vi "전체 Test.vi"() -> ()   [LabVIEW 2020]
uses:
  <vilib>/userDefined/High Color/IMAQdx.ctl
  <vilib>/Utility/miscctls.llb/LVPointTypeDef.ctl
  <vilib>/DAQmx/read.llb/DAQmx Read (Analog 1D Wfm NChan NSamp).vi
  <vilib>/Analysis/baseanly.llb/Mean (DBL).vi
  <vilib>/DAQmx/create/channels.llb/DAQmx Create Channel (AI-Voltage-Basic).vi
  <vilib>/DAQmx/configure/timing.llb/DAQmx Timing (Sample Clock).vi
  <vilib>/DAQmx/miscellaneous.llb/DAQmx Fill In Error Info.vi
  <vilib>/Analysis/NI_AALBase.lvlib
  <vilib>/vision/driver/NI_Vision_Acquisition_Software.lvlib
  <vilib>/Utility/file.llb/Write Delimited Spreadsheet (DBL).vi
panel:
  out "거리":waveform(dbl)(graph)
  out "기울기":waveform(dbl)[](graph)
  out "가속도":waveform(dbl)(graph)
  out "Image":T1(plugin-control)
  in  "data out":string
  out "CNN Result":string[](array[string])
  in  "CNN Data Save Path":path
  out "Capture Image":T1(plugin-control) caption="Captuer Image"
  out "Softmax Result":string
  in  "Softmax Data Save Path":path
  in  "정지":bool
  in  "측정 시작":bool
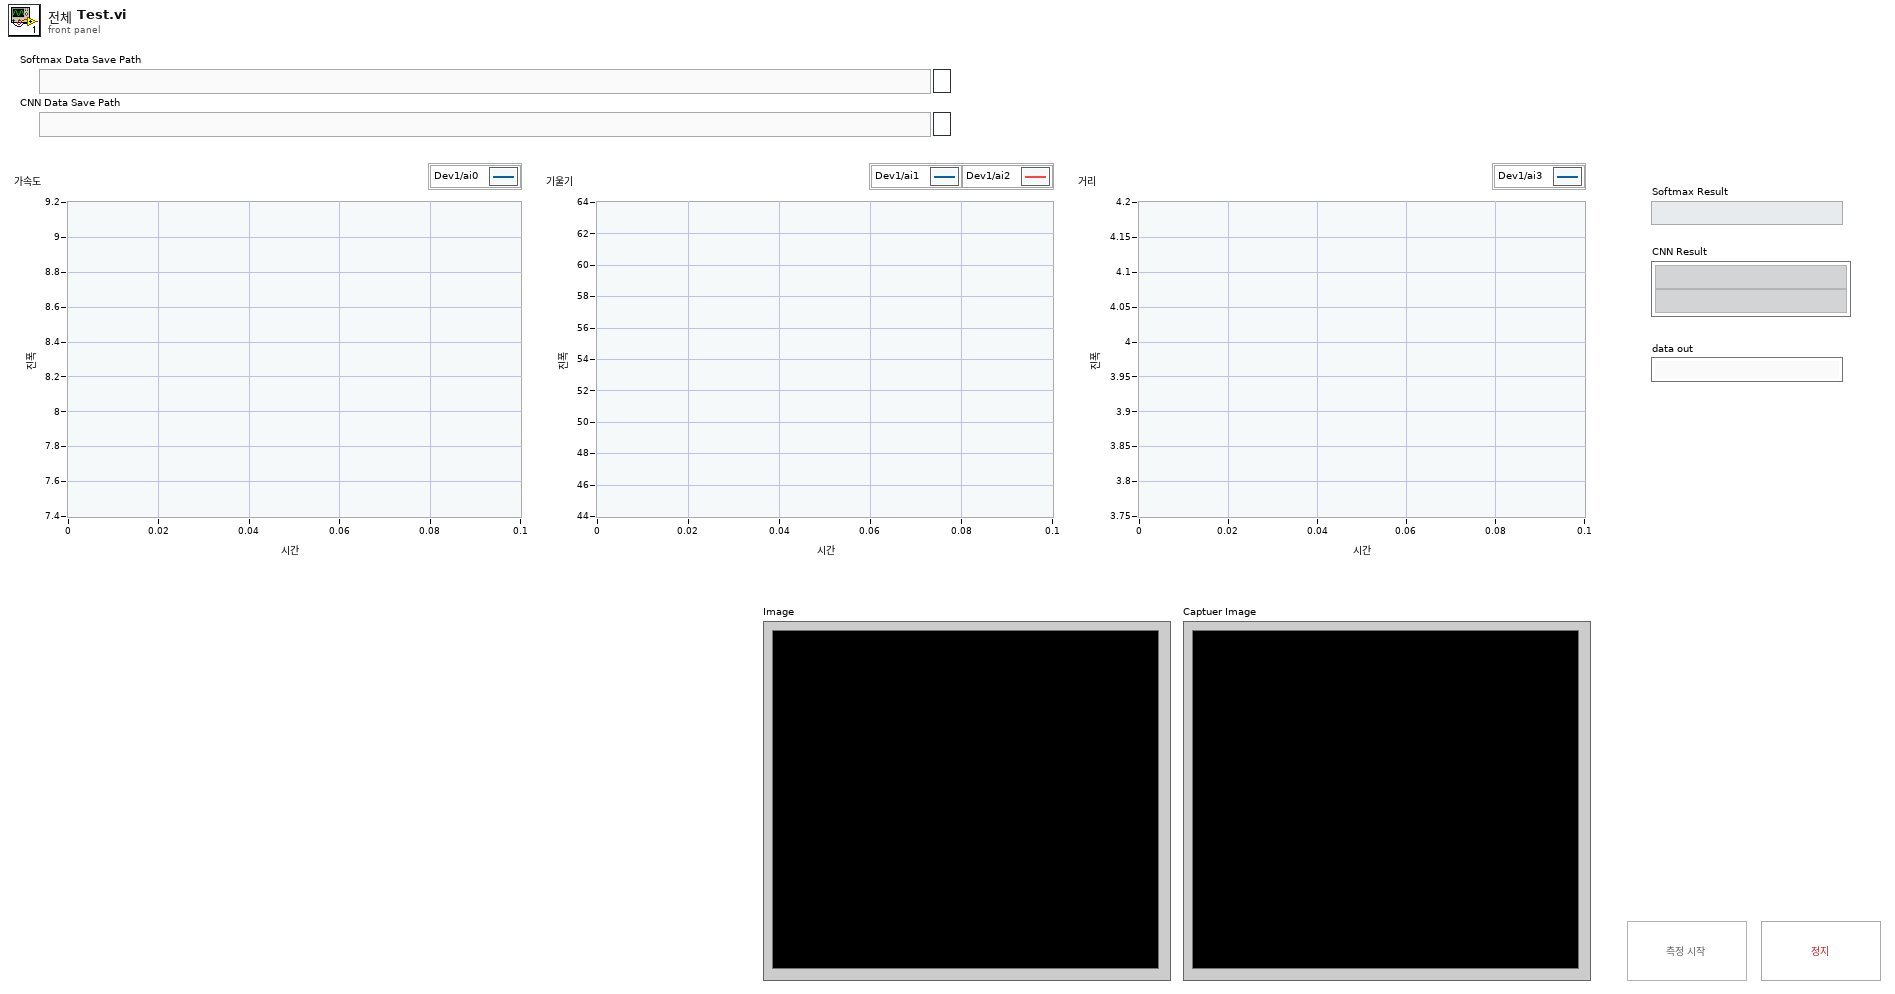
[diagram p1: front panel]
types:
  T1 = typedef "IMAQ Image.ctl" = refnum<image>
  T2 = typedef "Image Type" = u32
  T3 = typedef "IMAQdx.ctl" = refnum<k21>
  T4 = enum8{"Enabled", "Disabled", "Disabled and Grayed Out"}
  T5 = typedef "LVPointTypeDef.ctl" = cluster{"Horizontal":i16, "Vertical":i16}
  T6 = cluster{"queue out":refnum<queue>, "queue out":refnum<queue>}
  T7 = enum16{"Standard", "Buffered", "CRLF", "Immediate"}
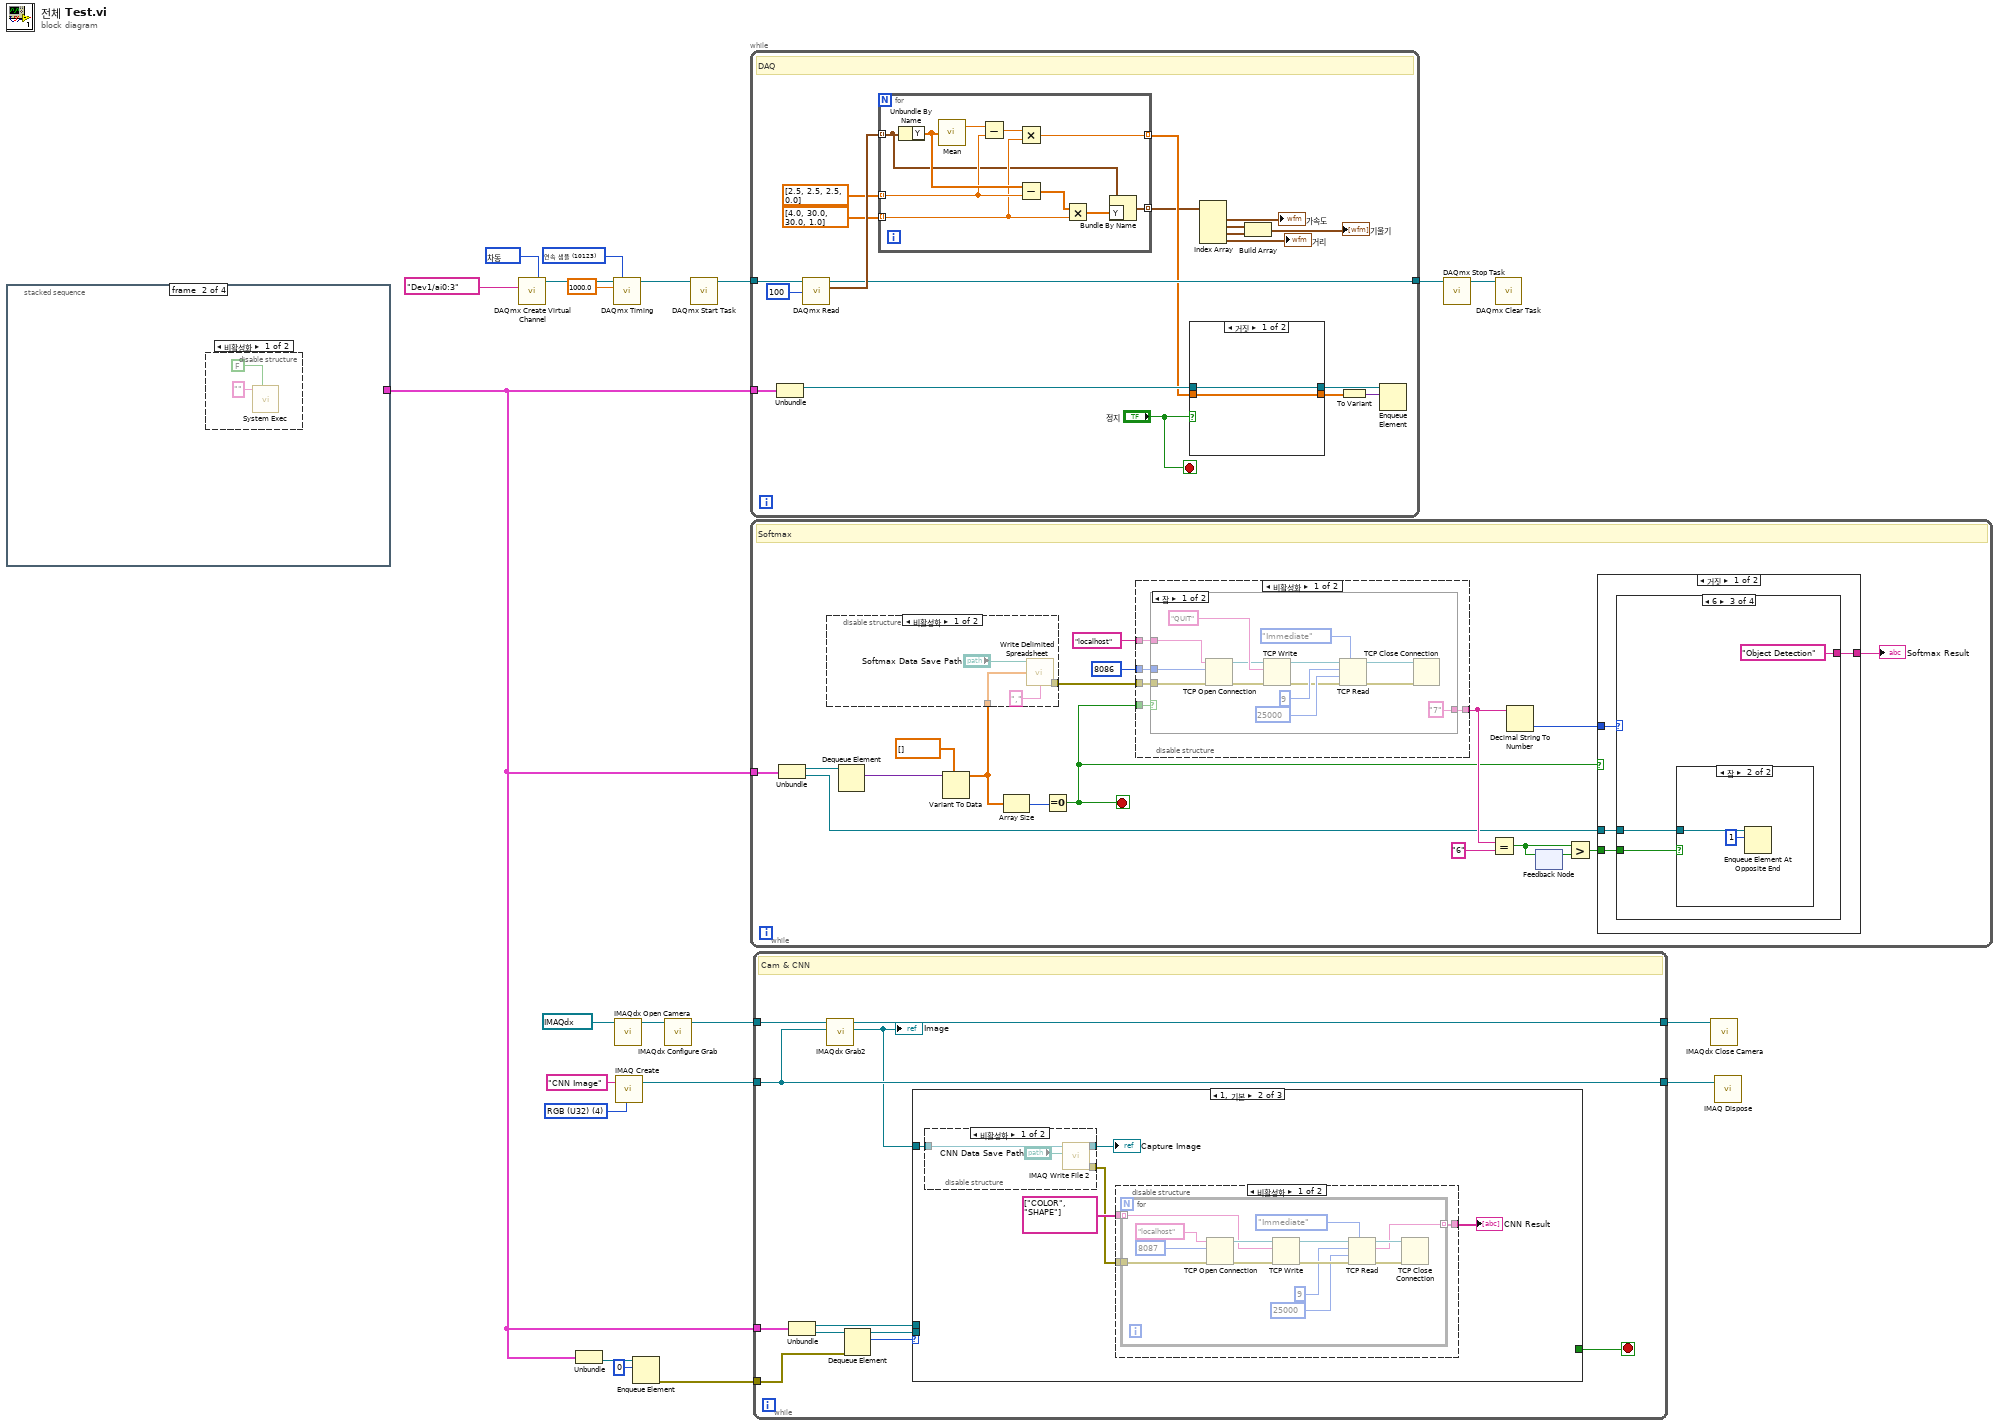
[diagram p0: block diagram]
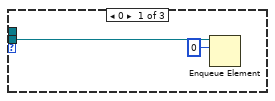
[diagram p2: hidden frame]
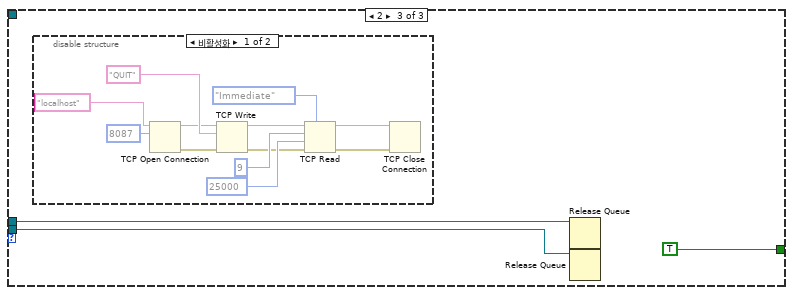
[diagram p5: hidden frame]
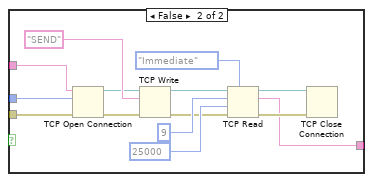
[diagram p8: hidden frame]
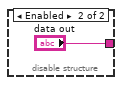
[diagram p9: hidden frame]
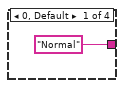
[diagram p10: hidden frame]
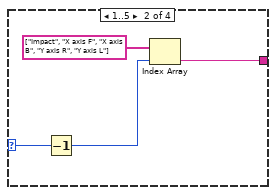
[diagram p11: hidden frame]
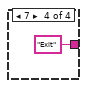
[diagram p13: hidden frame]
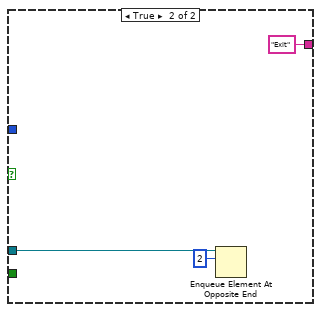
[diagram p14: hidden frame]
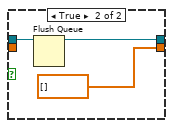
[diagram p15: hidden frame]
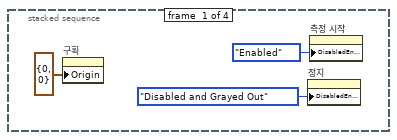
[diagram p16: hidden frame]
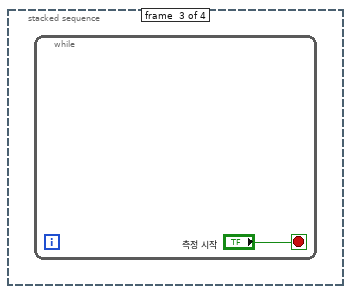
[diagram p18: hidden frame]
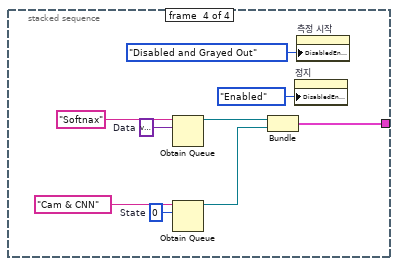
[diagram p19: hidden frame]
diagram:
  w8 = T2 4 items=["Grayscale (U8)", "Grayscale (I16)", "Grayscale (SGL)", "Complex (CSG)", "RGB (U32)", "HSL (U32)", "RGB (U64)", "Grayscale (U16)"] ("Image Type")
  w16 = 10123 items=["유한 샘플"=10178, "연속 샘플"=10123, "하드웨어 타이밍에 의한 단일 포인트"=12522] ("sample mode")
  w20 = 10106 items=["기본"=-1, "RSE"=10083, "NRSE"=10078, "차동"=10106, "유사 차동"=12529] ("input terminal configuration")
  n1 = stacked-sequence {
    tunnel: [_ _ _ w30] -> w3
    frame #0 {
      n2 = property on="구획" class="Pane"("Origin"=T5 {"Horizontal"=0, "Vertical"=0} ("원점")) -> ()  [unwired: 2 in, 2 out]
      n3 = property on="정지" class="Bool"("DisabledEnum"=T4."Disabled and Grayed Out" ("비활성화")) -> ()  [unwired: 2 in, 2 out]
      n4 = property on="측정 시작" class="Bool"("DisabledEnum"=T4."Enabled" ("비활성화")) -> ()  [unwired: 2 in, 2 out]
    }
    frame #1 {
      n5 = disable-structure shown="비활성화" {
        frame Disabled {
          n6 = call <vilib>:"System Exec.vi"("wait until completion? (T)"=FALSE, "command line"="") -> ()  [unwired: 6 in, 4 out]
        }
        frame Enabled {
        }
      }
    }
    frame #2 {
      n7 = while {
        stop <- "측정 시작" stop-if-true
      }
    }
    frame #3 {
      w33 = 0  # State
      w34 = variant  # Data
      n8 = Obtain Queue(name (unnamed)="Softnax" ("이름(이름없음)"), element data type=w34) -> (queue out=w32:refnum<queue>)  [unwired: 3 in, 2 out]
      n9 = Obtain Queue(name (unnamed)="Cam & CNN" ("이름(이름없음)"), element data type=w33) -> (queue out=w31:refnum<queue>)  [unwired: 3 in, 2 out]
      n10 = Bundle("queue out"=w32, "queue out"=w31) -> (w30:T6)  [unwired: 1 in]
      n11 = property on="정지" class="Bool"("DisabledEnum"=T4."Enabled" ("비활성화")) -> ()  [unwired: 2 in, 2 out]
      n12 = property on="측정 시작" class="Bool"("DisabledEnum"=T4."Disabled and Grayed Out" ("비활성화")) -> ()  [unwired: 2 in, 2 out]
    }
  }
  n13 = call-poly <vilib>:"DAQmx Create Virtual Channel.vi"("input terminal configuration"=w20, "physical channels"=tag "Dev1/ai0:3") -> ("task out"=w19:refnum<k21>)  [unwired: 12 in, 1 out]
  n14 = Unbundle(w3) -> ("queue out"=w2:refnum<queue>)  [unwired: 1 out]
  n15 = call-poly <vilib>:"DAQmx Timing.vi"("task/channels in"=w19, "sample mode"=w16, "rate"=1000.0) -> ("task out"=w18:refnum<k21>)  [unwired: 11 in, 1 out]
  n16 = call <vilib>:"IMAQdx Open Camera.vi"("Session In"=T3 "cam2") -> ("Session Out"=w11:T3)  [unwired: 9 in, 1 out]
  n17 = call "IMAQ Create"("Image Name"="CNN Image", "Image Type"=w8) -> ("New Image"=w7:T1)  [unwired: 3 in, 1 out]
  n18 = Enqueue Element(queue=w2, element=0 ("원소")) -> (error out=w1:errorcluster)  [unwired: 2 in, 2 out]
  n19 = call <vilib>:"IMAQdx Configure Grab.vi"("Session In"=w11) -> ("Session Out"=w10:T3)  [unwired: 9 in, 1 out]
  n20 = call <vilib>:"DAQmx Start Task.vi"("task/channels in"=w18) -> ("task out"=w17:refnum<k21>)  [unwired: 13 in, 1 out]
  n21 = while {
    tunnel: w3 -> [w55]
    tunnel: w17 -> [w51]
    tunnel: [w48] -> w14
    stop <- "정지" stop-if-true
    # "DAQ"
    n22 = Unbundle(w55) -> ("queue out"=w53:refnum<queue>)  [unwired: 1 out]
    n23 = call-poly <vilib>:"DAQmx Read.vi"("task/channels in"=w51, "number of samples per channel"=100) -> ("task out"=w48:refnum<k21>, "data"=w49:waveform(dbl)[])  [unwired: 11 in, 1 out]
    n24 = for {
      tunnel: w49 -> [w57] mode=indexing
      tunnel: dbl[] [2.5, 2.5, 2.5, 0.0] -> [w61] mode=indexing
      tunnel: dbl[] [4.0, 30.0, 30.0, 1.0] -> [w59] mode=indexing
      tunnel: [w63] -> w45 mode=indexing
      tunnel: [w56] -> w42 mode=indexing
      n25 = Unbundle By Name(w57) -> ("Y"=w62:dbl[])
      n26 = call-poly <vilib>:"Mean.vi"("X"=w62) -> ("mean"=w65:dbl)  [unwired: 1 out]
      n27 = Subtract(x=w65, y=w61) -> (x-y=w64:dbl)
      n28 = Multiply(x=w64, y=w59) -> (x*y=w63:dbl)
      n29 = Subtract(x=w62, y=w61) -> (x-y=w60:dbl[])
      n30 = Multiply(x=w60, y=w59) -> (x*y=w58:dbl[])
      n31 = Bundle By Name(cluster=w57, "Y"=w58) -> (w56:waveform(dbl))
    }
    n32 = case shown="거짓" "정지" {
      tunnel: w53 -> [w67 w70]
      tunnel: [w67 w69] -> w52
      tunnel: w45 -> [w66 _]
      tunnel: [w66 dbl[] []] -> w43
      frame False {
      }
      frame True {
        n33 = Flush Queue(queue=w70) -> (queue out=w69:refnum<queue>)  [unwired: 1 in, 2 out]
      }
    }
    n34 = Index Array(array=w42) -> (element #1=→"가속도":waveform(dbl), element #2=w41:waveform(dbl), element #3=w40:waveform(dbl), element #4=→"거리":waveform(dbl))  [unwired: 4 in]
    n35 = Build Array(w41, w40) -> (→"기울기":waveform(dbl)[])
    n36 = To Variant(anything=w43) -> (Variant=w44:variant)
    n37 = Enqueue Element(queue=w52, element=w44) -> ()  [unwired: 2 in, 3 out]
  }
  n38 = while {
    tunnel: w3 -> [w88]
    stop <- w73 stop-if-true
    # "Softmax"
    n39 = Unbundle(w88) -> ("queue out"=w87:refnum<queue>, "queue out"=w74:refnum<queue>)
    n40 = Dequeue Element(queue=w87) -> (element=w86:variant)  [unwired: 2 in, 3 out]
    n41 = Variant To Data(type=dbl[] [], Variant=w86) -> (data=w84:dbl[])  [unwired: 1 in, 1 out]
    n42 = disable-structure shown="비활성화" {
      disable-tunnel: w84 -> [w92 _]
      disable-tunnel: [w89 _] -> w83
      frame Disabled {
        n43 = call-poly <vilib>:"Write Delimited Spreadsheet.vi"("file path (dialog if empty)"="Softmax Data Save Path", "1D data"=w92, "delimiter (\\t)"="," ("delimiter (\\t)")) -> ("error out"=w89:errorcluster)  [unwired: 11 in, 1 out]
      }
      frame Enabled {
      }
    }
    n44 = Array Size(array=w84) -> (size(s)=w85:i32)
    n45 = Equal To 0?(x=w85) -> (x = 0?=w73:bool)
    n46 = disable-structure shown="비활성화" {
      disable-tunnel: w83 -> [w97 _]
      disable-tunnel: "localhost" ("address") -> [w96 _]
      disable-tunnel: u16 8086 ("원격 포트 또는 서비스 이름") -> [w95 _]
      disable-tunnel: [w94 "data out"] -> w76
      disable-tunnel: w73 -> [w93 _]
      frame Disabled {
        n47 = case shown="참" w93 {
          tunnel: w97 -> [w104 w118]
          tunnel: w96 -> [w100 w114]
          tunnel: w95 -> [w99 w113]
          tunnel: ["7" ("data out") w112] -> w94
          frame True {
            n48 = TCP Open Connection(address=w100, remote port or service name=w99, error in (no error)=w104) -> (connection ID=w106:refnum<k5>, error out=w105:errorcluster)  [unwired: 2 in]
            n49 = TCP Write(connection ID=w106, data in="QUIT", error in (no error)=w105) -> (connection ID out=w108:refnum<k5>, error out=w107:errorcluster)  [unwired: 1 in, 1 out]
            n50 = TCP Read(connection ID=w108, bytes to read=9, error in (no error)=w107, 7:T7."Immediate" ("모드(standard)"), 9:25000 ("timeout ms (25000)")) -> (connection ID out=w102:refnum<k5>, error out=w101:errorcluster)  [unwired: 1 out]
            n51 = TCP Close Connection(connection ID=w102, error in (no error)=w101) -> ()  [unwired: 1 in, 2 out]
          }
          frame False {
            n52 = TCP Open Connection(address=w114, remote port or service name=w113, error in (no error)=w118) -> (connection ID=w120:refnum<k5>, error out=w119:errorcluster)  [unwired: 2 in]
            n53 = TCP Write(connection ID=w120, data in="SEND", error in (no error)=w119) -> (connection ID out=w122:refnum<k5>, error out=w121:errorcluster)  [unwired: 1 in, 1 out]
            n54 = TCP Read(connection ID=w122, bytes to read=9, error in (no error)=w121, 7:T7."Immediate" ("모드(standard)"), 9:25000 ("timeout ms (25000)")) -> (connection ID out=w116:refnum<k5>, data out=w112:string, error out=w115:errorcluster)
            n55 = TCP Close Connection(connection ID=w116, error in (no error)=w115) -> ()  [unwired: 1 in, 2 out]
          }
        }
      }
      frame Enabled {
      }
    }
    n56 = Equal?(x=w76, y="6") -> (x = y?=w78:bool)
    n57 = Decimal String To Number(string=w76) -> (number=w75:i32)  [unwired: 2 in, 1 out]
    n58 = feedback #1() -> (w79:bool)  [unwired: 1 in]
    n59 = feedback-in #1(w78) -> ()
    n60 = Greater?(x=w78, y=w79) -> (0:w77:bool)
    n61 = case shown="거짓" w73 {
      tunnel: w77 -> [w130 _]
      tunnel: w75 -> [w129 _]
      tunnel: w74 -> [w128 w144]
      tunnel: [w127 "Exit"] -> w72
      frame False {
        n62 = case shown="6" w129 {
          selector: w129 -> [_ w133 _ _]
          tunnel: w130 -> [_ _ w136 _]
          tunnel: ["Normal" w134 "Object Detection" "Exit"] -> w127
          tunnel: w128 -> [_ _ w137 _]
          frame 0, Default {
          }
          frame 1..5 {
            n63 = Decrement(x=w133) -> (x-1=w132:i32)
            n64 = Index Array(array=string[] ["Impact", "X axis F", "X axis B", "Y axis R", "Y axis L"], index=w132) -> (element=w134:string)
          }
          frame 6 {
            n65 = case shown="참" w136 {
              tunnel: w137 -> [_ w140]
              frame False {
              }
              frame True {
                n66 = Enqueue Element At Opposite End(queue=w140, element=1 ("원소")) -> ()  [unwired: 2 in, 3 out]
              }
            }
          }
          frame 7 {
          }
        }
      }
      frame True {
        n67 = Enqueue Element At Opposite End(queue=w144, element=2 ("원소")) -> ()  [unwired: 2 in, 3 out]
      }
    }
    "Softmax Result" <- w72
  }
  n68 = while {
    tunnel: w3 -> [w155]
    tunnel: w10 -> [w152]
    tunnel: w7 -> [w147]
    tunnel: [w151] -> w6
    tunnel: [w147] -> w5
    tunnel: w1 -> [w145]
    stop <- w148 stop-if-true
    # "Cam & CNN"
    n69 = Unbundle(w155) -> ("queue out"=w150:refnum<queue>, "queue out"=w154:refnum<queue>)
    n70 = call <vilib>:"IMAQdx Grab2.vi"("Image In"=w147, "Session In"=w152) -> ("Image Out"=w146:T1, "Session Out"=w151:T3)  [unwired: 6 in, 2 out]
    "Image" <- w146
    n71 = Dequeue Element(queue=w154, error in (no error)=w145) -> (queue out=w149:refnum<queue>, element=w153:i32)  [unwired: 1 in, 2 out]
    n72 = case shown="1, 기본" w153 {
      tunnel: w146 -> [_ w162 _]
      tunnel: w150 -> [_ _ w187]
      tunnel: w149 -> [w157 _ w186]
      tunnel: [_ _ TRUE] -> w148
      frame 0 {
        n73 = Enqueue Element(queue=w157, element=0 ("원소")) -> ()  [unwired: 2 in, 3 out]
      }
      frame 1, Default {
        n74 = disable-structure shown="비활성화" {
          disable-tunnel: w162 -> [w166 w167]
          disable-tunnel: [w164 w167] -> w161
          disable-tunnel: [w163 _] -> w159
          frame Disabled {
            n75 = call-poly "IMAQ Write File 2"("File Path"="CNN Data Save Path", "Image"=w166) -> ("error out"=w163:errorcluster, "Image Out (duplicate)"=w164:T1)  [unwired: 8 in]
          }
          frame Enabled {
          }
        }
        "Capture Image" <- w161
        n76 = disable-structure shown="비활성화" {
          disable-tunnel: string[] ["COLOR", "SHAPE"] ("데이터 입력") -> [w170 _]
          disable-tunnel: w159 -> [w169 _]
          disable-tunnel: [w168 _] -> w158
          frame Disabled {
            n77 = for {
              tunnel: w169 -> [w184]
              tunnel: [w172] -> w168 mode=indexing
              tunnel: w170 -> [w171] mode=indexing
              n78 = TCP Open Connection(address="localhost", remote port or service name=u16 8087 ("원격 포트 또는 서비스 이름"), error in (no error)=w184) -> (connection ID=w179:refnum<k5>, error out=w180:errorcluster)  [unwired: 2 in]
              n79 = TCP Write(connection ID=w179, data in=w171, error in (no error)=w180) -> (connection ID out=w176:refnum<k5>, error out=w177:errorcluster)  [unwired: 1 in, 1 out]
              n80 = TCP Read(connection ID=w176, bytes to read=9, error in (no error)=w177, 7:T7."Immediate" ("모드(standard)"), 9:25000 ("timeout ms (25000)")) -> (connection ID out=w181:refnum<k5>, data out=w172:string, error out=w182:errorcluster)
              n81 = TCP Close Connection(connection ID=w181, error in (no error)=w182) -> ()  [unwired: 1 in, 2 out]
            }
          }
          frame Enabled {
          }
        }
        "CNN Result" <- w158
      }
      frame 2 {
        n82 = disable-structure shown="비활성화" {
          frame Disabled {
            n83 = TCP Open Connection(address="localhost" ("주소"), remote port or service name=u16 8087 ("원격 포트 또는 서비스 이름")) -> (connection ID=w194:refnum<k5>, error out=w193:errorcluster)  [unwired: 3 in]
            n84 = TCP Write(connection ID=w194, data in="QUIT", error in (no error)=w193) -> (connection ID out=w196:refnum<k5>, error out=w195:errorcluster)  [unwired: 1 in, 1 out]
            n85 = TCP Read(connection ID=w196, bytes to read=9, error in (no error)=w195, 7:T7."Immediate" ("모드(standard)"), 9:25000 ("timeout ms (25000)")) -> (connection ID out=w191:refnum<k5>, error out=w190:errorcluster)  [unwired: 1 out]
            n86 = TCP Close Connection(connection ID=w191, error in (no error)=w190) -> ()  [unwired: 1 in, 2 out]
          }
          frame Enabled {
          }
        }
        n87 = Release Queue(queue=w187) -> ()  [unwired: 2 in, 3 out]
        n88 = Release Queue(queue=w186) -> ()  [unwired: 2 in, 3 out]
      }
    }
  }
  n89 = call <vilib>:"DAQmx Stop Task.vi"("task/channels in"=w14) -> ("task out"=w13:refnum<k21>)  [unwired: 13 in, 1 out]
  n90 = call <vilib>:"DAQmx Clear Task.vi"("task in"=w13) -> ()  [unwired: 14 in, 1 out]
  n91 = call <vilib>:"IMAQdx Close Camera.vi"("Session In"=w6) -> ()  [unwired: 10 in, 1 out]
  n92 = call "IMAQ Dispose"("Image"=w5) -> ()  [unwired: 5 in, 1 out]
